vi "configure scope.vi"(0 "instrument handle":refnum<k15>, 1 "Voltage Channel Range":dbl(ring)=200.0 items=["200V"=200.0, "700V"=700.0, "1400V"=1400.0], 2 "Voltage Channel Input Offset":dbl(ring) items=["+500"=500.0, "0"=0.0, "-500"=-500.0], 3 "Voltage vertical coupling":T1=1 items=["AC", "DC", "Ground"], 7 "Sample Rate":dbl=10000000.0 min=1.0 max=10000000.0 format="%_3p S/s", 11 "error in":errorcluster, 12 "Current Channel Range":dbl(ring)=10.0 items=["10A"=10.0, "35A"=35.0, "70A"=70.0], 13 "Current Channel Input Offset":dbl(ring) items=["+25"=25.0, "0"=0.0, "-25"=-25.0], 14 "Current vertical coupling":T1=1 items=["AC", "DC", "Ground"]) -> (4 "instrument handle out":refnum<k15>, 6 "Voltage Channel Input Impedance":string, 10 "Current Channel Input Impedence":string, 15 "error out":errorcluster)   [LabVIEW 2018]
uses:
  <instrlib>/niScope/Controls/niScope vertical coupling.ctl
  <instrlib>/niScope/Configure/Trigger/niScope Configure Trigger Immediate.vi
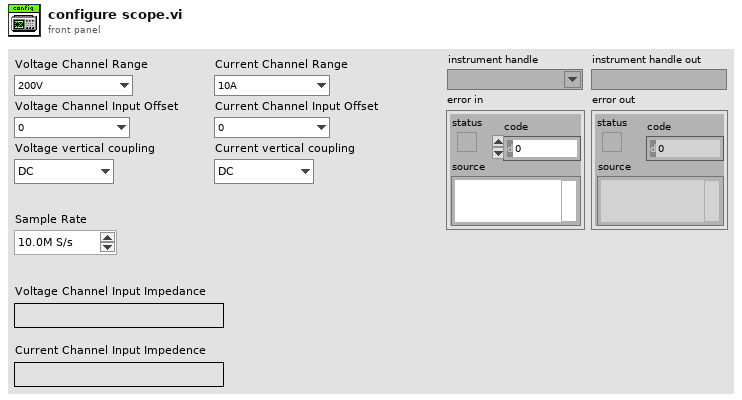
[diagram p1: front panel]
types:
  T1 = typedef "niScope vertical coupling.ctl" = i32
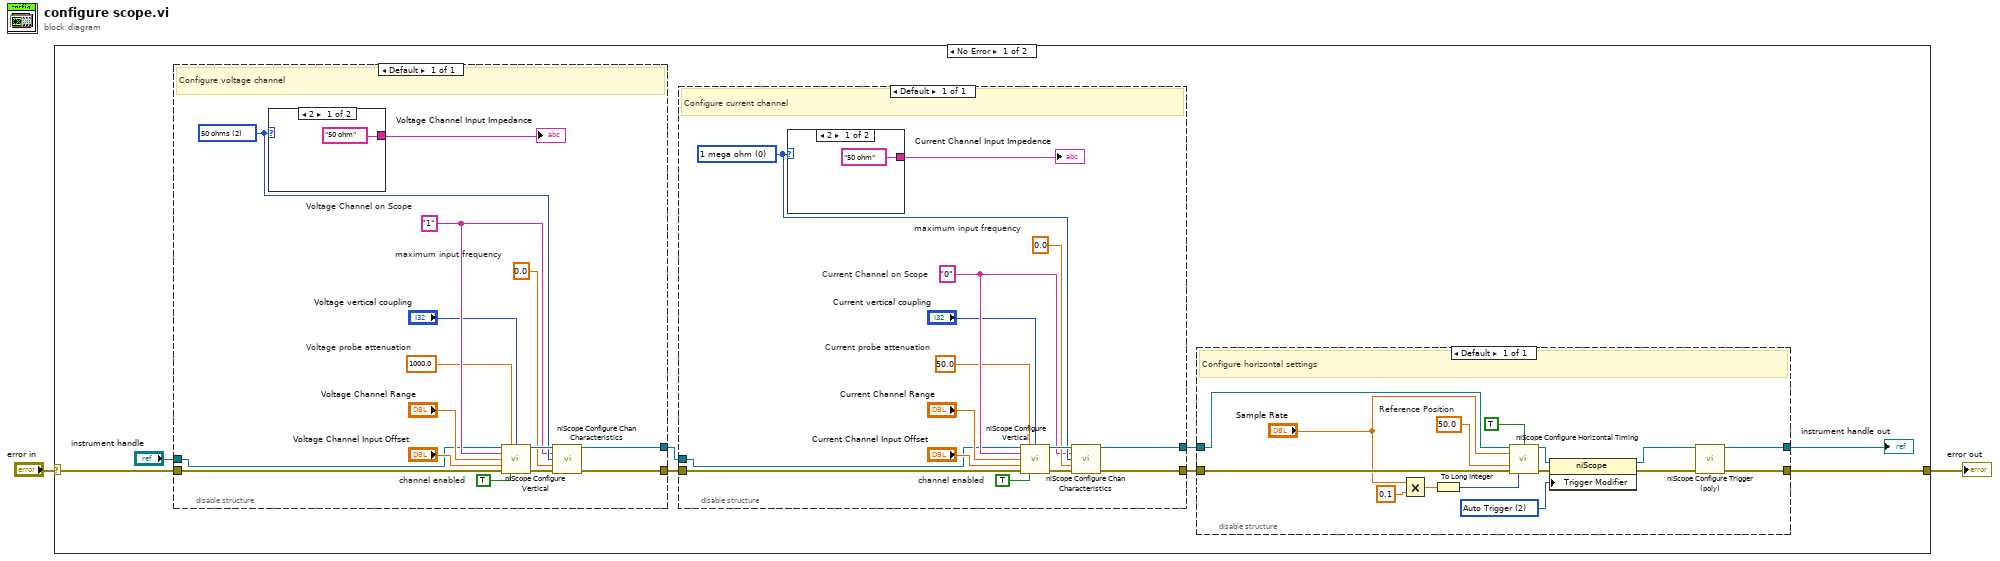
[diagram p0: block diagram]
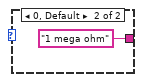
[diagram p2: hidden frame]
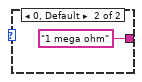
[diagram p3: hidden frame]
diagram:
  n1 = case shown="No Error" "error in" {
    selector: "error in" -> [w10 w60]
    tunnel: [w3 w60] -> w2
    frame No Error {
      n2 = disable-structure shown="Default" {
        disable-tunnel: [w29] -> w9
        disable-tunnel: w10 -> [w28]
        disable-tunnel: [w27] -> w8
        disable-tunnel: "instrument handle" -> [w26]
        frame Enabled {
          w37 = 0.0  # maximum input frequency
          w31 = 1000.0  # Voltage probe attenuation
          w32 = "1"  # Voltage Channel on Scope
          w36 = u32 2 items=["1 mega ohm"=0, "50 ohms"=2] ("input impedance")
          w35 = TRUE  # channel enabled
          # "Configure voltage channel"
          n3 = case shown="2" w36 {
            tunnel: ["50 ohm" ("Voltage Channel Input Impedence") "1 mega ohm" ("Voltage Channel Input Impedence")] -> w38
            frame 2 {
            }
            frame 0, Default {
            }
          }
          "Voltage Channel Input Impedance" <- w38
          n4 = call <instrlib>:"niScope Configure Vertical.vi"("instrument handle"=w26, "probe attenuation"=w31, "vertical coupling"="Voltage vertical coupling", "channels"=w32, "vertical range"="Voltage Channel Range", "vertical offset"="Voltage Channel Input Offset", "error in"=w28, "channel enabled"=w35) -> ("instrument handle out"=w40:refnum<k15>, "error out"=w39:errorcluster)  [unwired: 6 out]
          n5 = call <instrlib>:"niScope Configure Chan Characteristics.vi"("instrument handle"=w40, "channels"=w32, "input impedance"=w36, "maximum input frequency"=w37, "error in"=w39) -> ("instrument handle out"=w27:refnum<k15>, "error out"=w29:errorcluster)  [unwired: 9 in]
        }
      }
      n6 = disable-structure shown="Default" {
        disable-tunnel: [w46] -> w5
        disable-tunnel: w9 -> [w45]
        disable-tunnel: w8 -> [w44]
        disable-tunnel: [w43] -> w6
        frame Enabled {
          w53 = 0.0  # maximum input frequency
          w47 = 50.0  # Current probe attenuation
          w52 = "0"  # Current Channel on Scope
          w49 = TRUE  # channel enabled
          w54 = u32 0 items=["1 mega ohm"=0, "50 ohms"=2] ("input impedance")
          # "Configure current channel"
          n7 = case shown="2" w54 {
            tunnel: ["50 ohm" ("Voltage Channel Input Impedence") "1 mega ohm" ("Voltage Channel Input Impedence")] -> w57
            frame 2 {
            }
            frame 0, Default {
            }
          }
          "Current Channel Input Impedence" <- w57
          n8 = call <instrlib>:"niScope Configure Vertical.vi"("instrument handle"=w44, "probe attenuation"=w47, "vertical coupling"="Current vertical coupling", "channels"=w52, "vertical range"="Current Channel Range", "vertical offset"="Current Channel Input Offset", "error in"=w45, "channel enabled"=w49) -> ("instrument handle out"=w56:refnum<k15>, "error out"=w55:errorcluster)  [unwired: 6 out]
          n9 = call <instrlib>:"niScope Configure Chan Characteristics.vi"("instrument handle"=w56, "channels"=w52, "input impedance"=w54, "maximum input frequency"=w53, "error in"=w55) -> ("instrument handle out"=w43:refnum<k15>, "error out"=w46:errorcluster)  [unwired: 9 in]
        }
      }
      n10 = disable-structure shown="Default" {
        disable-tunnel: w6 -> [w16]
        disable-tunnel: w5 -> [w15]
        disable-tunnel: [w14] -> w4
        disable-tunnel: [w13] -> w3
        frame Enabled {
          w23 = 50.0  # Reference Position
          w20 = 2 items=["None"=1, "Auto Trigger"=2] ("Trigger Modifier")
          # "Configure horizontal settings"
          n11 = Multiply(x="Sample Rate", y=0.1) -> (x*y=w24:dbl)
          n12 = To Long Integer(number=w24) -> (32bit integer=w17:i32)
          n13 = call <instrlib>:"niScope Configure Horizontal Timing.vi"("instrument handle"=w16, "enforce realtime"=TRUE ("Enforce Realtime"), "min sample rate"="Sample Rate", "reference position"=w23, "error in"=w15, "min record length"=w17) -> ("instrument handle out"=w22:refnum<k15>, "error out"=w21:errorcluster)  [unwired: 8 in]
          n14 = property on="Property Node" class="niScope"(reference=w22, error in=w21, "Trigger Modifier"=w20) -> (reference out=w19:refnum<k15>, error out=w18:errorcluster)
          n15 = call-poly <instrlib>:"niScope Configure Trigger (poly).vi"("instrument handle"=w19, "error in"=w18) -> ("instrument handle out"=w14:refnum<k15>, "error out"=w13:errorcluster)  [unwired: 12 in]
        }
      }
      "instrument handle out" <- w4
    }
    frame Error {
    }
  }
  "error out" <- w2
